vi "Untitled 1.vi"() -> ()   [LabVIEW 2015]
panel:
  out "Numeric 3":dbl
  in  "error in (no error)":errorcluster
  in  "stop 2":bool
  out "Numeric 2":dbl
  out "Beats per Minute":dbl
  out "Numeric":dbl
  in  "stop":bool
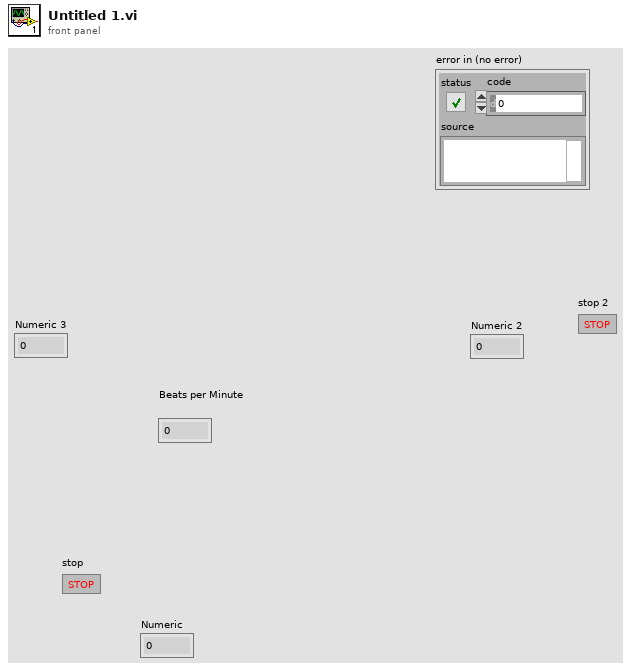
[diagram p1: front panel]
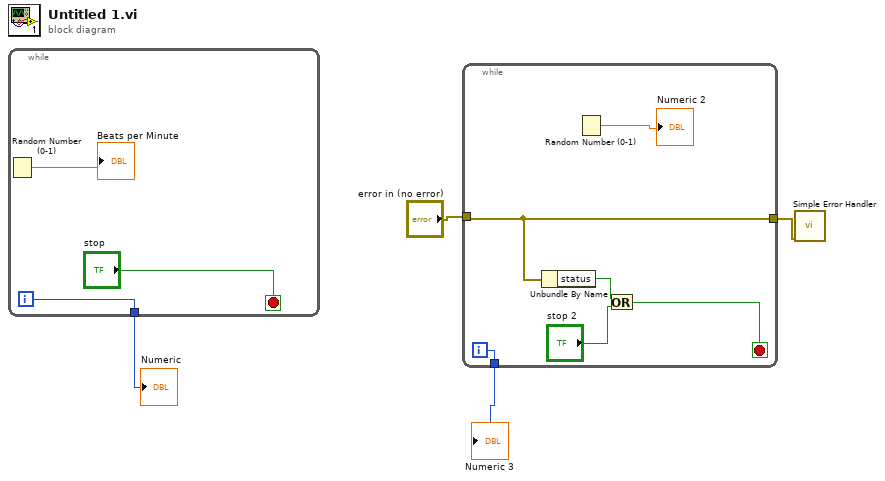
[diagram p0: block diagram]
diagram:
  n1 = while {
    tunnel: [w5] -> w4
    i -> [w5]
    stop <- "stop" stop-if-true
    n2 = Random Number (0-1)() -> (number: 0 to 1=→"Beats per Minute":dbl)
  }
  "Numeric" <- w4
  n3 = while {
    tunnel: "error in (no error)" -> [w12]
    tunnel: [w12] -> w2
    tunnel: [w8] -> w1
    i -> [w8]
    stop <- w9 stop-if-true
    n4 = Unbundle By Name(w12) -> ("status"=w10:bool)
    n5 = Random Number (0-1)() -> (number: 0 to 1=→"Numeric 2":dbl)
    n6 = Or(x=w10, y="stop 2") -> (x .or. y?=w9:bool)
  }
  "Numeric 3" <- w1
  n7 = call <vilib>:"Simple Error Handler.vi"("error in (no error)"=w2) -> ()  [unwired: 4 in, 5 out]
